vi "Autonomous.vi"() -> ()   [LabVIEW 2018]
uses:
  <vilib>/Studica/Studica Toolkit/Background/DIO Channel.ctl
  <vilib>/Studica/Studica Toolkit/Background/Mxp Selection.ctl
  <vilib>/robotics/Steering/Steering Frame/Apply Steering Frame Velocity to Motors.vi
  <vilib>/robotics/Steering/Steering Frame/Get Steering Frame Velocity from Motors.vi
  <vilib>/robotics/Steering/Steering Frame/NI_Robotics_Steering Frame.lvclass
  <vilib>/Studica/Studica Blackhawk/Blackhawk.lvlib
  <vilib>/Studica/Studica Toolkit/Background/I2C Channel.ctl
  <vilib>/Studica/Studica Toolkit/NavX/NavX.lvlib
panel:
  in  "Start Location (X,Y)":cluster{"X":dbl, "Y":dbl, "Theta":dbl}
  in  "Workstations":T1
  in  "Movement Accuracy":dbl=0.05 format="%#_13g"
  in  "SetPoints":T2
  in  "y":dbl=0.158982 format="%#_13g"
  in  "Speed":dbl[](array[numeric])=[-0.058732406271419055, -0.1288548481696414, 1.6548681508478632e-17]
  out "Hoist Height":dbl
  in  "CC's":T3={"CC 1"={"Ball #1"="Yellow", "Ball #2"="Red"}}
  in  "Wanted Location":dbl[](array[numeric])=[0.0, 0.0, 0.0]
  in  "Yellow Ball Bin":cluster{"X":dbl, "Y":dbl, "Theta":dbl}={"X"=-5.0, "Y"=5.0, "Theta"=0.0}
  in  "Orange Ball Bin":cluster{"X":dbl, "Y":dbl, "Theta":dbl}={"X"=5.0, "Y"=-5.0, "Theta"=0.0}
  in  "Red Ball Bin":cluster{"X":dbl, "Y":dbl, "Theta":dbl}={"X"=-5.0, "Y"=-5.0, "Theta"=0.0}
  in  "Blue Ball Bin":cluster{"X":dbl, "Y":dbl, "Theta":dbl}={"X"=5.0, "Y"=5.0, "Theta"=0.0}
  in  "CC 6":cluster{"X":dbl, "Y":dbl, "Theta":dbl}
  in  "CC 5":cluster{"X":dbl, "Y":dbl, "Theta":dbl}
  in  "CC 4":cluster{"X":dbl, "Y":dbl, "Theta":dbl}
  in  "CC 3":cluster{"X":dbl, "Y":dbl, "Theta":dbl}
  in  "CC 2":cluster{"X":dbl, "Y":dbl, "Theta":dbl}
  in  "CC 1":cluster{"X":dbl, "Y":dbl, "Theta":dbl}
  in  "Main Operation":string="Put Balls on CC"
  in  "Location PID":T4(array[cluster])=[{"proportional gain (Kc)"=10.0, "integral time (Ti, min)"=0.0, "derivative time (Td, min)"=0.0}, {"proportional gain (Kc)"=10.0, "integral time (Ti, min)"=0.0, "derivative time (Td, min)"=0.0}, {"proportional gain (Kc)"=10.0, "integral time (Ti, min)"=0.0, "derivative time (Td, min)"=0.0}] {"integral time (Ti, min)" min=0.0 step=0.0001}
  out "Estimated Robot Location":dbl[](array[numeric])=[0.036942802500546636, 0.08104996047957719, -1.0409154186309538e-17]
  out "Yaw":dbl
  in  "Wanted Rotation Angle":dbl[](array[numeric])=[0.0] format="%.2f"
  in  "NavX PID gains":T4(array[cluster])=[{"proportional gain (Kc)"=0.15, "integral time (Ti, min)"=0.0, "derivative time (Td, min)"=0.003}] {"integral time (Ti, min)" min=0.0 step=0.0001}
  in  "Hoist Setpoint (Height)":dbl
  in  "Button LED":bool
  out "estimated steering frame velocity":dbl[](array[numeric])
  in  "Green LED":bool=TRUE
  in  "Red LED":bool
  in  "Program Done?":bool
  in  "Robot Model":string(combo)="3-wheeled"
  in  "Reset Encoders":bool
  in  "StopMotors":bool
  in  "Stop Program":bool
  in  "Robot Facing":i16=4
  out "PID-Output":dbl[](array[numeric])=[-0.01145281922292672, 0.027486766135024127, -0.016033946912097405, -0.016033946912097405]
  in  "PID gains":T4(array[cluster])=[{"proportional gain (Kc)"=1.3, "integral time (Ti, min)"=0.004, "derivative time (Td, min)"=0.0}, {"proportional gain (Kc)"=1.3, "integral time (Ti, min)"=0.004, "derivative time (Td, min)"=0.0}, {"proportional gain (Kc)"=1.3, "integral time (Ti, min)"=0.004, "derivative time (Td, min)"=0.0}] {"proportional gain (Kc)" step=0.01; "integral time (Ti, min)" min=0.0 step=0.0001; "derivative time (Td, min)" step=0.0001}
  out "Actual-SpeedList":dbl[](array[numeric])
  in  "Linear Hoist":dbl(slide) scale=-1.0..1.0
  # "Configuration"
  # "LED's"
  # "Speed related shit"
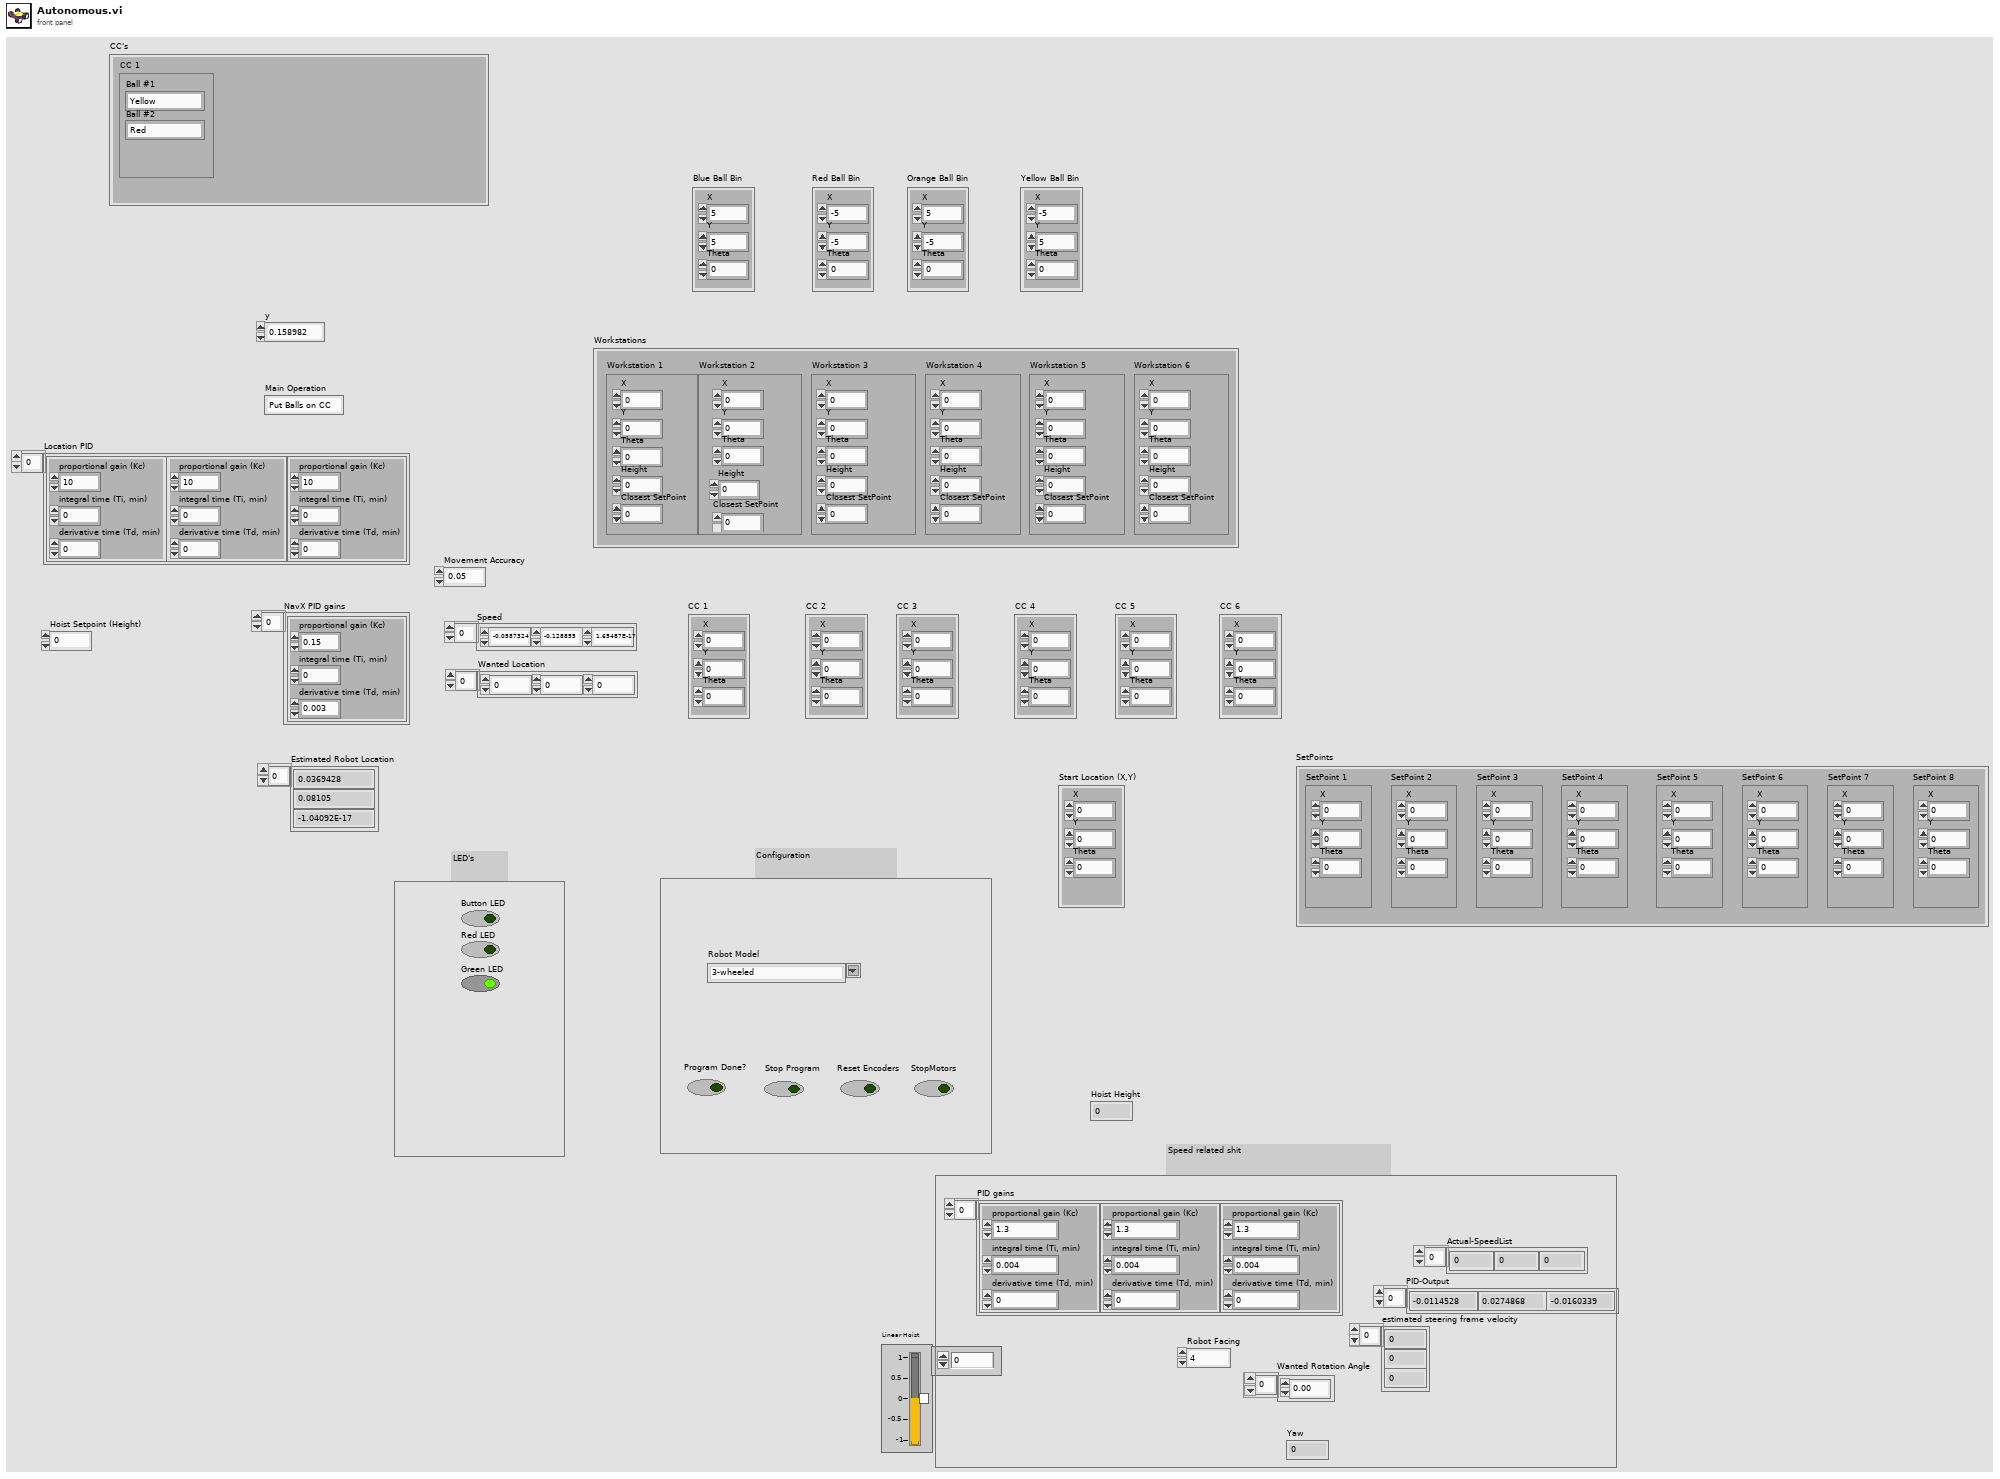
[diagram p1: front panel]
types:
  T1 = cluster{"Workstation 1":cluster{"X":dbl, "Y":dbl, "Theta":dbl, "Height":dbl, "Closest SetPoint":dbl}, "Workstation 2":cluster{"X":dbl, "Y":dbl, "Theta":dbl, "Height":dbl, "Closest SetPoint":dbl}, "Workstation 3":cluster{"X":dbl, "Y":dbl, "Theta":dbl, "Height":dbl, "Closest SetPoint":dbl}, "Workstation 4":cluster{"X":dbl, "Y":dbl, "Theta":dbl, "Height":dbl, "Closest SetPoint":dbl}, "Workstation 5":cluster{"X":dbl, "Y":dbl, "Theta":dbl, "Height":dbl, "Closest SetPoint":dbl}, "Workstation 6":cluster{"X":dbl, "Y":dbl, "Theta":dbl, "Height":dbl, "Closest SetPoint":dbl}}
  T2 = cluster{"SetPoint 1":cluster{"X":dbl, "Y":dbl, "Theta":dbl}, "SetPoint 2":cluster{"X":dbl, "Y":dbl, "Theta":dbl}, "SetPoint 3":cluster{"X":dbl, "Y":dbl, "Theta":dbl}, "SetPoint 4":cluster{"X":dbl, "Y":dbl, "Theta":dbl}, "SetPoint 5":cluster{"X":dbl, "Y":dbl, "Theta":dbl}, "SetPoint 6":cluster{"X":dbl, "Y":dbl, "Theta":dbl}, "SetPoint 7":cluster{"X":dbl, "Y":dbl, "Theta":dbl}, "SetPoint 8":cluster{"X":dbl, "Y":dbl, "Theta":dbl}}
  T3 = cluster{"CC 1":cluster{"Ball #1":string, "Ball #2":string}}
  T4 = cluster{"proportional gain (Kc)":dbl, "integral time (Ti, min)":dbl, "derivative time (Td, min)":dbl}[]
  T5 = typedef "DIO Channel.ctl" = enum16{"Not Connected", "A/DIO1", "A/DIO2", "A/DIO3", "A/DIO4", "A/DIO5", "A/DIO6", "A/DIO7", "A/DIO13", "B/DIO1", "B/DIO2", "B/DIO3", "B/DIO4", "B/DIO5", "B/DIO6", "B/DIO7", "B/DIO13", "C/DIO0", "C/DIO1", "C/DIO2", "C/DIO3", "C/DIO4", "C/DIO5", "C/DIO6", "C/DIO7"}
  T6 = typedef "Mxp Selection.ctl" = enum16{"MXP A", "MXP B"}
  T7 = typedef "I2C Channel.ctl" = enum16{"Not Connected", "A", "B"}
  T8 = cluster{"DIO Channel":T5, "FPGA VI Reference Out":refnum<k20>}
  T9 = typedef "I2C.lvlib/I2C Reference.ctl" = cluster{"myRIO Reference":T10, "I2C Channels Enum":T14, "I2C Configuration":T15}
  T10 = typedef "myRIO Generic Hardware Reference.ctl" = cluster{"myRIO Model":T11, "myRIO Hardware Reference":T12}
  T11 = typedef "Hardware Version Enum.ctl" = enum16{"Unknown", "myRIO-1900", "myRIO-1950", "roboRIO", "NI ELVIS RIO CM", "ELVIS III"}
  T12 = typedef "myRIO v1.0 Reference.ctl" = cluster{"Generic FPGA Reference":T13, "Allow multiple opens":bool}
  T13 = typedef "Generic FPGA Reference.ctl" = refnum<k20>
  T14 = typedef "I2C Channels Enum.ctl" = enum16{"Not Connected", "A/I2C", "B/I2C", "I2C/I2C"}
  T15 = typedef "I2C.lvlib/I2C Configuration.ctl" = cluster{"I2C Transfer Rate":T16}
  T16 = typedef "I2C.lvlib/I2C Transfer Rate.ctl" = enum16{"Standard mode (100 kbps)", "Fast mode (400 kbps)"}
  T17 = cluster{"I2C Ref Out":cluster{"I2C Channel":T7, "FPGA VI Reference Out":refnum<k20>}, "Connected":bool, "Slave Address (7-bit)":u8, "Registry":u8[]}
  T18 = cluster{"Yaw":dbl, "Roll":dbl, "Pitch":dbl, "Heading":dbl, "Fused Heading":dbl}
  T19 = cluster{"X":dbl, "Y":dbl, "Theta":dbl, "Height":dbl, "Closest SetPoint":dbl}[]
  T20 = cluster{"X":dbl, "Y":dbl, "Theta":dbl, "Height":dbl, "Closest SetPoint":dbl}
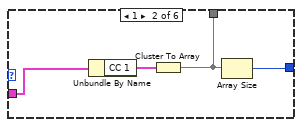
[diagram p3: hidden frame]
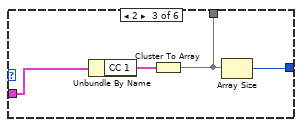
[diagram p4: hidden frame]
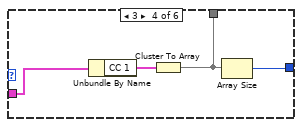
[diagram p5: hidden frame]
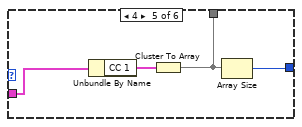
[diagram p6: hidden frame]
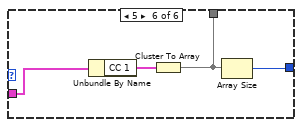
[diagram p7: hidden frame]
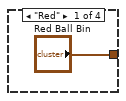
[diagram p8: hidden frame]
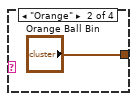
[diagram p9: hidden frame]
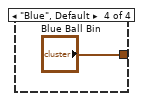
[diagram p10: hidden frame]
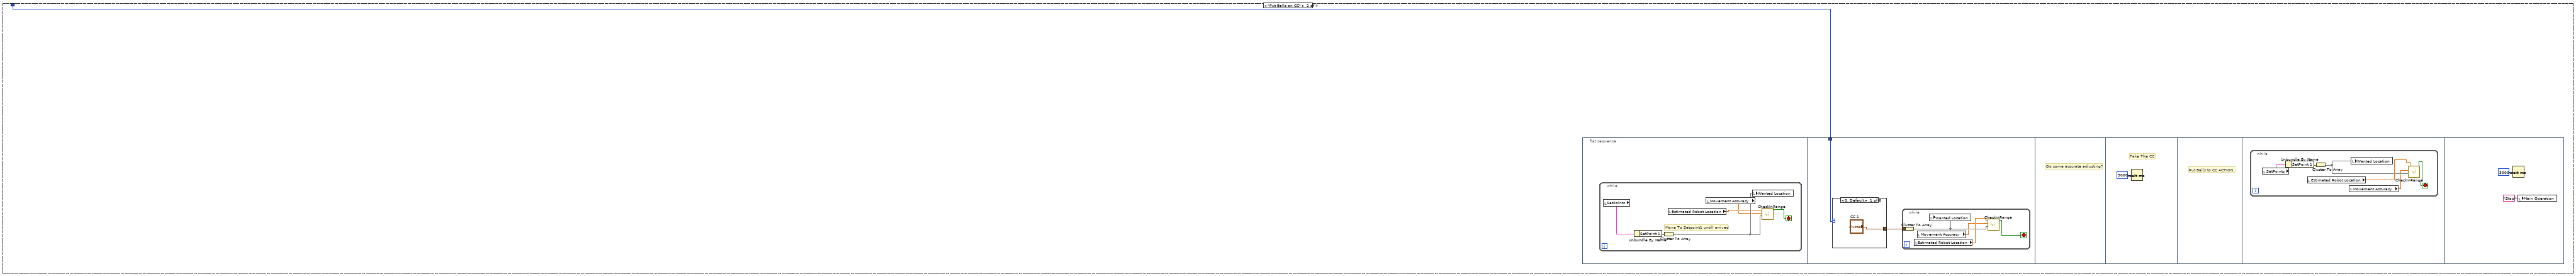
[diagram p12: hidden frame]
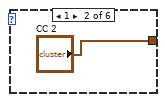
[diagram p13: hidden frame]
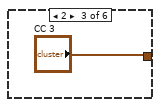
[diagram p14: hidden frame]
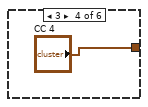
[diagram p15: hidden frame]
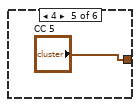
[diagram p16: hidden frame]
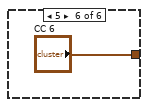
[diagram p17: hidden frame]
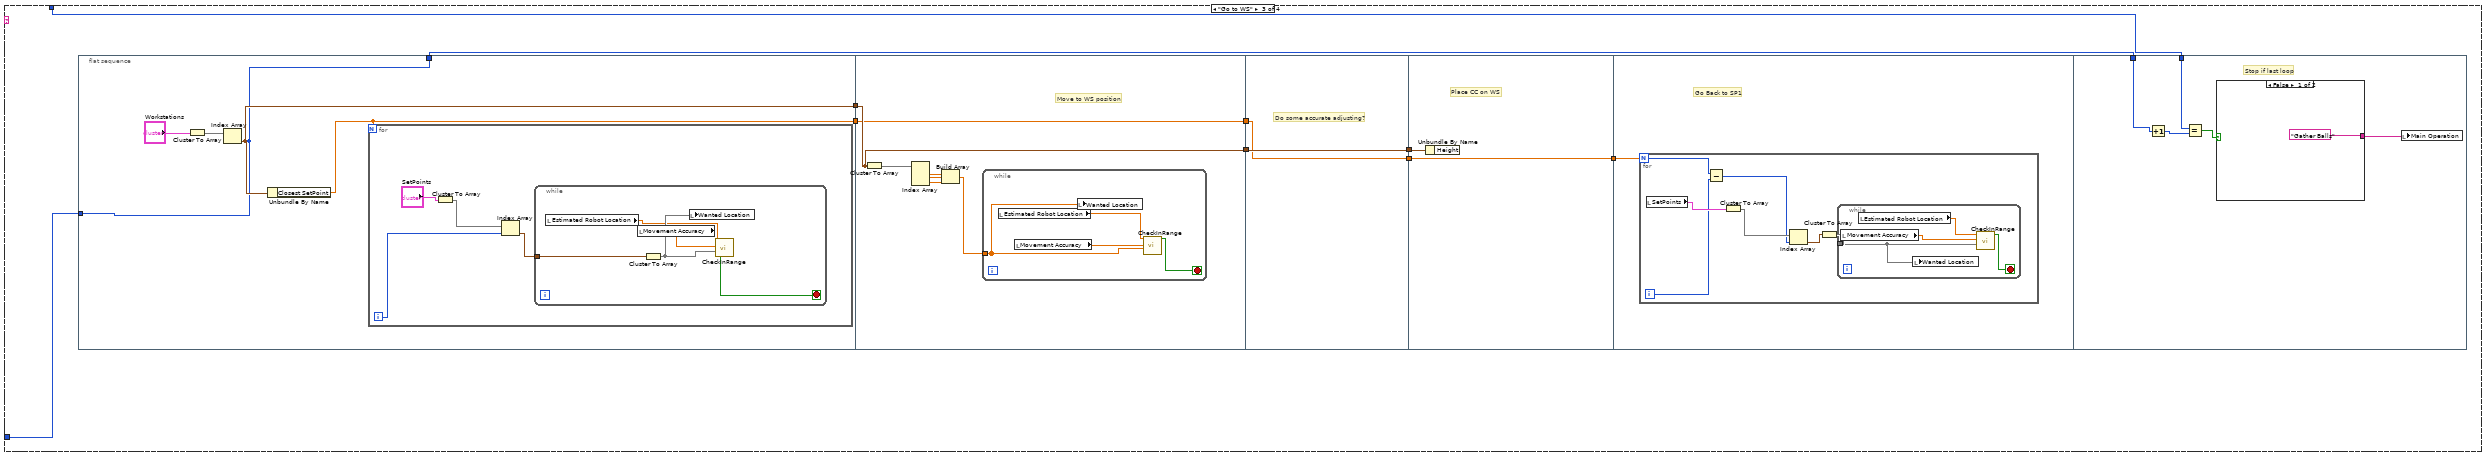
[diagram p18: hidden frame]
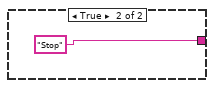
[diagram p19: hidden frame]
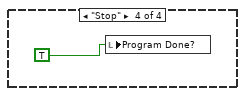
[diagram p20: hidden frame]
diagram:
  n1 = flat-sequence {
    frame #0 {
      # "Initialize"
      n2 = flat-sequence {
        frame #0 {
          w6 = FALSE ("StopMotors")
          w5 = FALSE ("StopMotors")
          n3 = flat-sequence {
            frame #0 {
              w7 = TRUE
              n4 = call <vilib>:"2 Encoders.vi"("Mxp Side"=Mxp_Selection."MXP A", "Reset Encoder 0"=w7, "Reset Encoder 1"=w7) -> ()  [unwired: 22 in, 3 out]
              n5 = call <vilib>:"2 Encoders.vi"("Mxp Side"=Mxp_Selection."MXP B", "Reset Encoder 0"=w7, "Reset Encoder 1"=w7) -> ()  [unwired: 22 in, 3 out]
            }
            frame #1 {
              w10 = FALSE
              n6 = call <vilib>:"2 Encoders.vi"("Mxp Side"=Mxp_Selection."MXP A", "Reset Encoder 0"=w10, "Reset Encoder 1"=w10) -> ()  [unwired: 22 in, 3 out]
              n7 = call <vilib>:"2 Encoders.vi"("Mxp Side"=Mxp_Selection."MXP B", "Reset Encoder 0"=w10, "Reset Encoder 1"=w10) -> ()  [unwired: 22 in, 3 out]
            }
          }
          n8 = local write "Button LED"(w6) -> ()
          n9 = local write "Red LED"(w6) -> ()
          n10 = local write "Green LED"(w6) -> ()
          n11 = local write "Program Done?"(w5) -> ()
          n12 = local write "Stop Program"(w5) -> ()
          n13 = local write "StopMotors"(w5) -> ()
          n14 = local write "Main Operation"("Gather Balls" ("Operation")) -> ()
        }
        frame #1 {
          n15 = disable-structure shown="Disabled" {
            frame Disabled {
              n16 = call <vilib>:"DIO Open.vi"("error in (no error)"=errorcluster {"status"=FALSE, "code"=0, "source"=""}, "DIO Channel"=DIO_Channel."C/DIO3") -> ("error out"=w16:errorcluster, "DIO Info Out"=w17:T8)  [unwired: 8 in]
              n17 = while {
                tunnel: w17 -> [w24]
                tunnel: w16 -> [w23]
                tunnel: [w22] -> w14
                tunnel: [w21] -> w13
                stop <- w19 stop-if-true
                # "Light Buttons LED"
                n18 = local write "Button LED"(TRUE ("Button LED")) -> ()
                n19 = call <vilib>:"C DIO Read.vi"("error in (no error)"=w23, "DIO Info In in"=w24) -> ("error out"=w21:errorcluster, "IN"=w19:bool, "DIO Info In out"=w22:T8)  [unwired: 7 in]
              }
              n20 = call <vilib>:"DIO Close.vi"("error in (no error)"=w13, "DIO Info In"=w14) -> ()  [unwired: 9 in, 1 out]
            }
            frame Enabled {
            }
          }
        }
        frame #2 {
          # "Light Green Led"
          n21 = local write "Button LED"(FALSE ("Button LED")) -> ()
          n22 = local write "Green LED"(TRUE ("Green LED")) -> ()
        }
      }
    }
    frame #1 {
      # "Loop for each cluster element(CC)"
      # "ENABLE THIS"
      # "Main"
      n23 = while {
        stop <- w205 stop-if-true
        n24 = local read "Estimated Robot Location"() -> (w199:dbl[])
        n25 = Multiply(x="Wanted Location", y="y") -> (x*y=w200:dbl[])
        n26 = Multiply(x=w199, y="y") -> (x*y=w197:dbl[])
        n27 = call "PID_array.vi"("output range"=cluster{"output high":dbl, "output low":dbl}[] [{"output high"=1.0, "output low"=-1.0}], "PID gains"="Location PID", "process variable"=w197, "setpoint"=w200) -> ("output"=w202:dbl[])  [unwired: 6 in, 1 out]
        n28 = local read "Stop Program"() -> (w205:bool)
        n29 = local write "Speed"(w202) -> ()
      }
      n30 = while {
        stop <- FALSE stop-if-true
        n31 = case shown="True" "Program Done?" {
          frame False {
          }
          frame True {
            # "Shut down Green Led"
            # "Light Red Led"
            n32 = local write "StopMotors"(TRUE ("StopMotors")) -> ()
            n33 = local write "Green LED"(FALSE ("Green LED")) -> ()
            n34 = local write "Red LED"(TRUE ("Red LED")) -> ()
          }
        }
      }
      n35 = disable-structure shown="Disabled" {
        frame Disabled {
          n36 = while {
            tunnel: tag "A/I2C" ("Channel Name") -> [w213]
            stop <- w212 stop-if-true
            n37 = call <vilib>:"Blackhawk i2c Open.vi"("error in (no error)"=errorcluster {"status"=FALSE, "code"=0, "source"=""}, "Channel Name"=w213) -> ("error out"=w209:errorcluster, "I2C Ref Out"=w210:T9)  [unwired: 2 in]
            n38 = local read "Stop Program"() -> (w212:bool)
            n39 = call <vilib>:"Blackhawk Relay.vi"("error in (no error)"=w209, "I2C Ref In"=w210) -> ("error out"=w207:errorcluster, "I2C Ref Out"=w208:T9)  [unwired: 8 in]
            n40 = call <vilib>:"Blackhawk DIO Read.vi"("I2C Ref In"=w208, "error in (no error)"=w207) -> ()  [unwired: 4 in, 3 out]
          }
        }
        frame Enabled {
        }
      }
      n41 = while {
        stop <- w222 stop-if-true
        n42 = local read "Hoist Height"() -> (w214:dbl)
        n43 = Multiply(x="Hoist Setpoint (Height)", y=45.382795) -> (x*y=w216:dbl)
        n44 = Multiply(x=w214, y=45.382795) -> (x*y=w220:dbl)
        n45 = Build Array(w216) -> (w217:dbl[])
        n46 = Build Array(w220) -> (w225:dbl[])
        n47 = call "PID_array.vi"("output range"=cluster{"output high":dbl, "output low":dbl}[] [{"output high"=1.0, "output low"=-1.0}], "process variable"=w225, "setpoint"=w217) -> ("output"=w224:dbl[])  [unwired: 7 in, 1 out]
        n48 = Index Array(array=w224) -> (element=w223:dbl)  [unwired: 1 in]
        n49 = local write "Linear Hoist"(w223) -> ()
        n50 = local read "Stop Program"() -> (w222:bool)
      }
      n51 = disable-structure shown="Disabled" {
        frame Disabled {
          n52 = while {
            tunnel: I2C_Channel."A" ("I2C Channel") -> [w195]
            stop <- w186 stop-if-true
            n53 = call <vilib>:"NavX Open.vi"("I2C Channel"=w195) -> ("NavX Info"=w196:T17)  [unwired: 9 in, 1 out]
            n54 = call <vilib>:"YRPHfH.vi"("NavX Info In"=w196) -> ("YRPHfH"=w191:T18)  [unwired: 3 in, 1 out]
            n55 = Unbundle By Name(w191) -> ("Yaw"=w190:dbl)
            "Yaw" <- w190
            n56 = Build Array(w190) -> (w189:dbl[])
            n57 = call "PID_array.vi"("output range"=cluster{"output high":dbl, "output low":dbl}[] [{"output high"=0.5, "output low"=-0.5}], "PID gains"="NavX PID gains", "process variable"=w189, "setpoint"="Wanted Rotation Angle") -> ("output"=w194:dbl[])  [unwired: 6 in, 1 out]
            n58 = Index Array(array=w194) -> (element=w187:dbl)  [unwired: 1 in]
            n59 = local read "Stop Program"() -> (w186:bool)
            n60 = local write item#-1(w187) -> ()
          }
        }
        frame Enabled {
        }
      }
      n61 = while "Motor Communication Loop" {
        stop <- w279 stop-if-true
        n62 = while {
          stop <- w280 stop-if-true
          n63 = case shown="False" "StopMotors" {
            frame False {
              n64 = while {
                tunnel: Mxp_Selection."MXP A" ("Mxp Side") -> [w295]
                tunnel: Mxp_Selection."MXP B" ("Mxp Side") -> [w294]
                stop <- w292 stop-if-true
                w291 = 50.0 ("Frequency [Hz]")
                n65 = local read "PID-Output"() -> (w293:dbl[])
                n66 = Index Array(array=w293) -> (element #1=w287:dbl, element #2=w286:dbl, element #3=w285:dbl)  [unwired: 3 in]
                n67 = local read "StopMotors"() -> (w292:bool)
                n68 = call <vilib>:"2 Motor.vi"("Mxp Side"=w294, "Speed M0"=w285, "Invert M0"=FALSE, "Speed M1"="Linear Hoist", "Frequency [Hz]"=w291) -> ()  [unwired: 14 in, 1 out]
                n69 = call <vilib>:"2 Motor.vi"("Mxp Side"=w295, "Speed M0"=w287, "Invert M0"=FALSE, "Speed M1"=w286, "Invert M1"=TRUE ("Invert M0"), "Frequency [Hz]"=w291) -> ()  [unwired: 13 in, 1 out]
              }
            }
            frame True {
              w296 = 50.0 ("Frequency [Hz]")
              w297 = 0.0 ("Speed M0")
              n70 = call <vilib>:"2 Motor.vi"("Mxp Side"=Mxp_Selection."MXP A", "Speed M0"=w297, "Speed M1"=w297, "Frequency [Hz]"=w296) -> ()  [unwired: 15 in, 1 out]
              n71 = call <vilib>:"2 Motor.vi"("Mxp Side"=Mxp_Selection."MXP B", "Speed M0"=w297, "Speed M1"=w297, "Frequency [Hz]"=w296) -> ()  [unwired: 15 in, 1 out]
            }
          }
          n72 = local read "Stop Program"() -> (w280:bool)
        }
        n73 = local read "Stop Program"() -> (w279:bool)
      }
      n74 = while "Wheel Velocity Measurement loop" {
        shift-right: [w235] -> _
        shift-left: _ -> [w254]
        shift-right: [w251] -> _
        shift-left: _ -> [w252]
        stop <- w247 stop-if-true
        w249 = 4.0 ("Wheel Diameter M1 (inches)")
        w257 = u32 1440 ("Ticks Per Rev M0")
        # "1440 * 3 * 10"
        # "Ticks travelled"
        # "Distance travelled\n(inch)"
        # "Wheel diam.\n(inch)"
        # "Ticks/rev"
        # "Ticks elapsed"
        # "Time elapsed"
        # "m/s"
        n75 = Wait (ms)(milliseconds to wait=u32 30) -> ()  [unwired: 1 out]
        n76 = call <vilib>:"2 Encoders.vi"("Mxp Side"=Mxp_Selection."MXP A", "Ticks Per Rev M0"=w257, "Wheel Diameter M0 (inches)"=w249, "Reset Encoder 0"="Reset Encoders", "Ticks Per Rev M1"=w257, "Wheel Diameter M1 (inches)"=w249, "Reset Encoder 1"="Reset Encoders") -> ("Distance M0 (inches)"=w258:dbl, "Distance M1 (inches)"=w259:dbl)  [unwired: 18 in, 1 out]
        n77 = call <vilib>:"2 Encoders.vi"("Mxp Side"=Mxp_Selection."MXP B", "Ticks Per Rev M0"=w257, "Wheel Diameter M0 (inches)"=w249, "Reset Encoder 0"="Reset Encoders", "Ticks Per Rev M1"=w257, "Wheel Diameter M1 (inches)"=w249, "Reset Encoder 1"="Reset Encoders") -> ("Distance M0 (inches)"=w260:dbl, "Distance M1 (inches)"=w250:dbl)  [unwired: 18 in, 1 out]
        n78 = Build Array(w258, w259, w260, w250) -> (w262:dbl[])
        n79 = local read "Robot Facing"() -> (w246:i16)
        n80 = Multiply(x=w262, y=2.54) -> (x*y=w236:dbl[])
        n81 = call "SteeringFrame.vi"() -> ("NI_Robotics_Steering Frame out"=w245:refnum<class "NI_Robotics_Steering Frame.lvclass">)  [unwired: 11 in]
        n82 = Multiply(x=w236, y=45.382795) -> (x*y=w235:dbl[])
        n83 = Tick Count (ms)() -> (millisecond timer value=w251:u32)
        n84 = case shown="2, Default" w246 {
          tunnel: w236 -> [w268 w274]
          tunnel: w245 -> [w267 w272]
          tunnel: [w265 w273] -> w243
          frame 4 {
            n85 = Build Array(0, 1, 2) -> (w266:i32[])
            n86 = call-poly <vilib>:"Get Velocity from Motors.vi"("wheel indexes"=w266, "ccw motor velocity states"=w268, "steering frame in"=w267) -> ("estimated steering frame velocity"=w265:dbl[])  [unwired: 6 in, 2 out]
          }
          frame 2, Default {
            n87 = Build Array(1, 2, 0) -> (w275:i32[])
            n88 = call-poly <vilib>:"Get Velocity from Motors.vi"("wheel indexes"=w275, "ccw motor velocity states"=w274, "steering frame in"=w272) -> ("estimated steering frame velocity"=w273:dbl[])  [unwired: 6 in, 2 out]
          }
        }
        n89 = Subtract(x=w235, y=w254) -> (x-y=w253:dbl[])
        n90 = Index Array(array=w235, index=3) -> (element=w233:dbl)
        n91 = Subtract(x=w251, y=w252) -> (x-y=w264:u32)
        n92 = Divide(x=w233, y=43.2) -> (x/y=→"Hoist Height":dbl)
        n93 = Cluster To Array(cluster="Start Location (X,Y)") -> (array=w244:dbl[])
        n94 = Divide(x=w253, y=w264) -> (x/y=w240:dbl[])
        n95 = Add(x=w244, y=w243) -> (x+y=→"Estimated Robot Location":dbl[])
        n96 = Divide(x=w240, y=10.0) -> (x/y=→"Actual-SpeedList":dbl[])
        n97 = local read "Stop Program"() -> (w247:bool)
      }
      n98 = Flatten To String(anything="CC's") -> (data string=w28:string)  [unwired: 3 in, 2 out]
      n99 = String Length(string=w28) -> (length=w27:i32)
      n100 = case shown="\"3-wheeled\", Default" "Robot Model" {
        frame "3-wheeled", Default {
          n101 = call "SteeringFrame.vi"() -> ("NI_Robotics_Steering Frame out"=w300:refnum<class "NI_Robotics_Steering Frame.lvclass">)  [unwired: 11 in]
          n102 = while "Motor Control Loop" {
            shift-right: [w313] -> _
            shift-left: w300 -> [w308]
            stop <- "Stop Program" stop-if-true
            # "Wanted speeds"
            # "PID-Adjusted\nOutput to Motors"
            # "Motor Velocity\nReal Time"
            # "PID Max. \nOutputRange"
            # "PID Setpoint"
            n103 = case shown="2, Default" "Robot Facing" {
              tunnel: w308 -> [w324 w335]
              tunnel: [w320 w331] -> w313
              tunnel: [w318 w328] -> w303
              tunnel: [w315 w326] -> w305
              tunnel: "Speed" -> [w314 w325]
              frame 2, Default {
                n104 = Build Array(1, 2, 0) -> (w317:i32[])
                n105 = local read "Actual-SpeedList"() -> (w316:dbl[])
                n106 = call-poly <vilib>:"Apply Velocity to Motors.vi"("wheel indexes"=w317, "steering frame velocity"=w314, "steering frame in"=w324) -> ("ccw motor velocity setpoints"=w318:dbl[], "steering frame out"=w319:refnum<class "NI_Robotics_Steering Frame.lvclass">)  [unwired: 4 in, 3 out]
                n107 = call-poly <vilib>:"Get Velocity from Motors.vi"("wheel indexes"=w317, "ccw motor velocity states"=w316, "steering frame in"=w319) -> ("estimated steering frame velocity"=w315:dbl[], "steering frame out"=w320:refnum<class "NI_Robotics_Steering Frame.lvclass">)  [unwired: 6 in, 1 out]
              }
              frame 4 {
                n108 = Build Array(0, 1, 2) -> (w329:i32[])
                n109 = local read "Actual-SpeedList"() -> (w327:dbl[])
                n110 = call-poly <vilib>:"Apply Velocity to Motors.vi"("wheel indexes"=w329, "steering frame velocity"=w325, "steering frame in"=w335) -> ("ccw motor velocity setpoints"=w328:dbl[], "steering frame out"=w330:refnum<class "NI_Robotics_Steering Frame.lvclass">)  [unwired: 4 in, 3 out]
                n111 = call-poly <vilib>:"Get Velocity from Motors.vi"("wheel indexes"=w329, "ccw motor velocity states"=w327, "steering frame in"=w330) -> ("estimated steering frame velocity"=w326:dbl[], "steering frame out"=w331:refnum<class "NI_Robotics_Steering Frame.lvclass">)  [unwired: 6 in, 1 out]
              }
            }
            "estimated steering frame velocity" <- w305
            n112 = local read "Actual-SpeedList"() -> (w306:dbl[])
            n113 = Divide(x=w303, y=40.0 ("Wheel Diameter M1 (inches)")) -> (x/y=w302:dbl[])
            n114 = call "PID_array.vi"("output range"=cluster{"output high":dbl, "output low":dbl}[] [{"output high"=1.0, "output low"=-1.0}, {"output high"=1.0, "output low"=-1.0}, {"output high"=1.0, "output low"=-1.0}, {"output high"=1.0, "output low"=-1.0}], "PID gains"="PID gains", "process variable"=w306, "setpoint"=w302) -> ("output"=→"PID-Output":dbl[])  [unwired: 6 in, 1 out]
          }
        }
      }
      n115 = for {
        N: w27 -> [w32]
        i -> [w31]
        # "Which CC is getting delivered"
        n116 = case shown="\"Gather Balls\", Default" "Main Operation" {
          tunnel: w32 -> [w36 w97 w126 _]
          tunnel: w31 -> [_ _ w128 _]
          frame "Gather Balls", Default {
            # "REMEMBER TO CHANGE THESE"
            n117 = local read "CC's"() -> (w37:T3)
            n118 = case shown="0, Default" w36 {
              tunnel: w37 -> [w41 w44 w48 w52 w56 w60]
              tunnel: [w38 w43 w47 w51 w55 w59] -> w35
              tunnel: [w39 w42 w46 w50 w54 w58] -> w34
              frame 0, Default {
                n119 = Unbundle By Name(w41) -> ("CC 1"=w40:cluster{"Ball #1":string, "Ball #2":string})
                n120 = Cluster To Array(cluster=w40) -> (array=w39:string[])
                n121 = Array Size(array=w39) -> (size(s)=w38:i32)
              }
              frame 1 {
                n122 = Unbundle By Name(w44) -> ("CC 1"=w45:cluster{"Ball #1":string, "Ball #2":string})
                n123 = Cluster To Array(cluster=w45) -> (array=w42:string[])
                n124 = Array Size(array=w42) -> (size(s)=w43:i32)
              }
              frame 2 {
                n125 = Unbundle By Name(w48) -> ("CC 1"=w49:cluster{"Ball #1":string, "Ball #2":string})
                n126 = Cluster To Array(cluster=w49) -> (array=w46:string[])
                n127 = Array Size(array=w46) -> (size(s)=w47:i32)
              }
              frame 3 {
                n128 = Unbundle By Name(w52) -> ("CC 1"=w53:cluster{"Ball #1":string, "Ball #2":string})
                n129 = Cluster To Array(cluster=w53) -> (array=w50:string[])
                n130 = Array Size(array=w50) -> (size(s)=w51:i32)
              }
              frame 4 {
                n131 = Unbundle By Name(w56) -> ("CC 1"=w57:cluster{"Ball #1":string, "Ball #2":string})
                n132 = Cluster To Array(cluster=w57) -> (array=w54:string[])
                n133 = Array Size(array=w54) -> (size(s)=w55:i32)
              }
              frame 5 {
                n134 = Unbundle By Name(w60) -> ("CC 1"=w61:cluster{"Ball #1":string, "Ball #2":string})
                n135 = Cluster To Array(cluster=w61) -> (array=w58:string[])
                n136 = Array Size(array=w58) -> (size(s)=w59:i32)
              }
            }
            n137 = for {
              N: w35 -> [w62]
              tunnel: w34 -> [w63]
              i -> [w64]
              n138 = flat-sequence {
                tunnel: w64 -> [w74]
                tunnel: w63 -> [w72]
                tunnel: w64 -> [w95]
                tunnel: w62 -> [w92]
                frame #0 {
                  n139 = while {
                    stop <- w67 stop-if-true
                    # "Move To Setpoint1 untill arrived"
                    n140 = local read "SetPoints"() -> (w65:T2)
                    n141 = Unbundle By Name(w65) -> ("SetPoint 1"=w66:cluster{"X":dbl, "Y":dbl, "Theta":dbl})
                    n142 = Cluster To Array(cluster=w66) -> (array=w69:dbl[])
                    n143 = local read "Estimated Robot Location"() -> (w68:dbl[])
                    n144 = local write "Wanted Location"(w69) -> ()
                    n145 = call "CheckInRange"("SetPoint"=w69, "y"="Movement Accuracy", "Estimated Robot Location"=w68) -> ("Boolean"=w67:bool)  [unwired: 8 in]
                  }
                }
                frame #1 {
                  n146 = Index Array(array=w72, index=w74) -> (element=w71:string)
                  n147 = case shown="\"Yellow\"" w71 {
                    tunnel: ["Red Ball Bin" "Orange Ball Bin" "Yellow Ball Bin" "Blue Ball Bin"] -> w73
                    frame "Red" {
                    }
                    frame "Orange" {
                    }
                    frame "Yellow" {
                    }
                    frame "Blue", Default {
                    }
                  }
                  n148 = while {
                    tunnel: w73 -> [w79]
                    stop <- w76 stop-if-true
                    n149 = Cluster To Array(cluster=w79) -> (array=w77:dbl[])
                    n150 = local read "Estimated Robot Location"() -> (w78:dbl[])
                    n151 = local read "Movement Accuracy"() -> (w75:dbl)
                    n152 = local write "Wanted Location"(w77) -> ()
                    n153 = call "CheckInRange"("SetPoint"=w77, "y"=w75, "Estimated Robot Location"=w78) -> ("Boolean"=w76:bool)  [unwired: 8 in]
                  }
                }
                frame #2 {
                  # "PICKUP BALL"
                  n154 = Wait (ms)(milliseconds to wait=u32 3000) -> ()  [unwired: 1 out]
                }
                frame #3 {
                  n155 = while {
                    stop <- w89 stop-if-true
                    n156 = local read "SetPoints"() -> (w86:T2)
                    n157 = local read "Estimated Robot Location"() -> (w90:dbl[])
                    n158 = Unbundle By Name(w86) -> ("SetPoint 1"=w88:cluster{"X":dbl, "Y":dbl, "Theta":dbl})
                    n159 = local read "Movement Accuracy"() -> (w85:dbl)
                    n160 = Cluster To Array(cluster=w88) -> (array=w87:dbl[])
                    n161 = local write "Wanted Location"(w87) -> ()
                    n162 = call "CheckInRange"("SetPoint"=w87, "y"=w85, "Estimated Robot Location"=w90) -> ("Boolean"=w89:bool)  [unwired: 8 in]
                  }
                }
                frame #4 {
                  n163 = Decrement(x=w92) -> (x-1=w93:i32)
                  n164 = Equal?(x=w95, y=w93) -> (x = y?=w94:bool)
                  n165 = case shown="True" w94 {
                    frame False {
                    }
                    frame True {
                      n166 = local write "Main Operation"("Put Balls on CC" ("Main Operation")) -> ()
                    }
                  }
                  n167 = Wait (ms)(milliseconds to wait=u32 3000) -> ()  [unwired: 1 out]
                }
              }
            }
          }
          frame "Put Balls on CC" {
            n168 = flat-sequence {
              tunnel: w97 -> [w104]
              frame #0 {
                n169 = while {
                  stop <- w101 stop-if-true
                  # "Move To Setpoint1 untill arrived"
                  n170 = local read "SetPoints"() -> (w100:T2)
                  n171 = Unbundle By Name(w100) -> ("SetPoint 1"=w99:cluster{"X":dbl, "Y":dbl, "Theta":dbl})
                  n172 = Cluster To Array(cluster=w99) -> (array=w103:dbl[])
                  n173 = local read "Estimated Robot Location"() -> (w102:dbl[])
                  n174 = local read "Movement Accuracy"() -> (w98:dbl)
                  n175 = local write "Wanted Location"(w103) -> ()
                  n176 = call "CheckInRange"("SetPoint"=w103, "y"=w98, "Estimated Robot Location"=w102) -> ("Boolean"=w101:bool)  [unwired: 8 in]
                }
              }
              frame #1 {
                n177 = case shown="0, Default" w104 {
                  tunnel: ["CC 1" "CC 2" "CC 3" "CC 4" "CC 5" "CC 6"] -> w105
                  frame 0, Default {
                  }
                  frame 1 {
                  }
                  frame 2 {
                  }
                  frame 3 {
                  }
                  frame 4 {
                  }
                  frame 5 {
                  }
                }
                n178 = while {
                  tunnel: w105 -> [w114]
                  stop <- w115 stop-if-true
                  n179 = Cluster To Array(cluster=w114) -> (array=w113:dbl[])
                  n180 = local read "Estimated Robot Location"() -> (w116:dbl[])
                  n181 = local read "Movement Accuracy"() -> (w112:dbl)
                  n182 = local write "Wanted Location"(w113) -> ()
                  n183 = call "CheckInRange"("SetPoint"=w113, "y"=w112, "Estimated Robot Location"=w116) -> ("Boolean"=w115:bool)  [unwired: 8 in]
                }
              }
              frame #2 {
                # "Do some accurate adjusting?"
              }
              frame #3 {
                # "Take The CC"
                n184 = Wait (ms)(milliseconds to wait=u32 3000) -> ()  [unwired: 1 out]
              }
              frame #4 {
                # "Put Balls to CC ACTION"
              }
              frame #5 {
                n185 = while {
                  stop <- w122 stop-if-true
                  n186 = local read "SetPoints"() -> (w119:T2)
                  n187 = Unbundle By Name(w119) -> ("SetPoint 1"=w121:cluster{"X":dbl, "Y":dbl, "Theta":dbl})
                  n188 = local read "Estimated Robot Location"() -> (w123:dbl[])
                  n189 = Cluster To Array(cluster=w121) -> (array=w120:dbl[])
                  n190 = local read "Movement Accuracy"() -> (w118:dbl)
                  n191 = local write "Wanted Location"(w120) -> ()
                  n192 = call "CheckInRange"("SetPoint"=w120, "y"=w118, "Estimated Robot Location"=w123) -> ("Boolean"=w122:bool)  [unwired: 8 in]
                }
              }
              frame #6 {
                n193 = Wait (ms)(milliseconds to wait=u32 3000) -> ()  [unwired: 1 out]
                n194 = local write "Main Operation"("Stop" ("Main Operation")) -> ()
              }
            }
          }
          frame "Go to WS" {
            n195 = flat-sequence {
              tunnel: [w138] -> w135
              tunnel: [w137] -> w132
              tunnel: w128 -> [w136]
              tunnel: [w136] -> w127
              tunnel: w135 -> [w151]
              tunnel: [w151] -> w134
              tunnel: w132 -> [w150]
              tunnel: [w150] -> w131
              tunnel: w134 -> [w162]
              tunnel: [w162] -> w133
              tunnel: w131 -> [w161]
              tunnel: [w161] -> w130
              tunnel: w133 -> [w164]
              tunnel: w130 -> [w163]
              tunnel: [w163] -> w129
              tunnel: w129 -> [w165]
              tunnel: w127 -> [w180]
              tunnel: w126 -> [w181]
              frame #0 {
                n196 = Cluster To Array(cluster="Workstations") -> (array=w140:T19)
                n197 = Index Array(array=w140, index=w136) -> (element=w138:T20)
                n198 = Unbundle By Name(w138) -> ("Closest SetPoint"=w137:dbl)
                n199 = for {
                  N: w137 -> [_]
                  i -> [w141]
                  n200 = Cluster To Array(cluster="SetPoints") -> (array=w143:cluster{"X":dbl, "Y":dbl, "Theta":dbl}[])
                  n201 = Index Array(array=w143, index=w141) -> (element=w142:cluster{"X":dbl, "Y":dbl, "Theta":dbl})
                  n202 = while {
                    tunnel: w142 -> [w146]
                    stop <- w149 stop-if-true
                    n203 = local read "Estimated Robot Location"() -> (w145:dbl[])
                    n204 = local read "Movement Accuracy"() -> (w147:dbl)
                    n205 = Cluster To Array(cluster=w146) -> (array=w148:dbl[])
                    n206 = local write "Wanted Location"(w148) -> ()
                    n207 = call "CheckInRange"("SetPoint"=w148, "y"=w147, "Estimated Robot Location"=w145) -> ("Boolean"=w149:bool)  [unwired: 8 in]
                  }
                }
              }
              frame #1 {
                # "Move to WS position"
                n208 = Cluster To Array(cluster=w151) -> (array=w156:dbl[])
                n209 = Index Array(array=w156) -> (element #1=w155:dbl, element #2=w154:dbl, element #3=w153:dbl)  [unwired: 3 in]
                n210 = Build Array(w155, w154, w153) -> (w152:dbl[])
                n211 = while {
                  tunnel: w152 -> [w158]
                  stop <- w160 stop-if-true
                  n212 = local read "Estimated Robot Location"() -> (w157:dbl[])
                  n213 = local read "Movement Accuracy"() -> (w159:dbl)
                  n214 = local write "Wanted Location"(w158) -> ()
                  n215 = call "CheckInRange"("SetPoint"=w158, "y"=w159, "Estimated Robot Location"=w157) -> ("Boolean"=w160:bool)  [unwired: 8 in]
                }
              }
              frame #2 {
                # "Do some accurate adjusting?"
              }
              frame #3 {
                # "Place CC on WS"
                n216 = Unbundle By Name(w164) -> ()  [unwired: 1 out]
              }
              frame #4 {
                # "Go Back to SP1"
                n217 = for {
                  N: w165 -> [w170]
                  i -> [w169]
                  n218 = local read "SetPoints"() -> (w171:T2)
                  n219 = Subtract(x=w170, y=w169) -> (x-y=w168:i32)
                  n220 = Cluster To Array(cluster=w171) -> (array=w172:cluster{"X":dbl, "Y":dbl, "Theta":dbl}[])
                  n221 = Index Array(array=w172, index=w168) -> (element=w167:cluster{"X":dbl, "Y":dbl, "Theta":dbl})
                  n222 = Cluster To Array(cluster=w167) -> (array=w166:dbl[])
                  n223 = while {
                    tunnel: w166 -> [w175]
                    stop <- w174 stop-if-true
                    n224 = local read "Movement Accuracy"() -> (w173:dbl)
                    n225 = local read "Estimated Robot Location"() -> (w176:dbl[])
                    n226 = local write "Wanted Location"(w175) -> ()
                    n227 = call "CheckInRange"("SetPoint"=w175, "y"=w173, "Estimated Robot Location"=w176) -> ("Boolean"=w174:bool)  [unwired: 8 in]
                  }
                }
              }
              frame #5 {
                # "Stop if last loop"
                n228 = Increment(x=w180) -> (x+1=w179:i32)
                n229 = Equal?(x=w181, y=w179) -> (x = y?=w178:bool)
                n230 = case shown="False" w178 {
                  tunnel: ["Gather Balls" "Stop"] -> w177
                  frame False {
                  }
                  frame True {
                  }
                }
                n231 = local write "Main Operation"(w177) -> ()
              }
            }
          }
          frame "Stop" {
            n232 = local write "Program Done?"(TRUE) -> ()
          }
        }
      }
    }
  }
  n233 = while "LED loop" {
    tunnel: DIO_Channel."C/DIO1" ("DIO Channel") -> [w345]
    tunnel: DIO_Channel."C/DIO0" ("DIO Channel") -> [w342]
    tunnel: DIO_Channel."C/DIO2" ("DIO Channel") -> [w336]
    stop <- w340 stop-if-true
    n234 = call <vilib>:"DIO Open.vi"("DIO Channel"=w345) -> ("error out"=w347:errorcluster, "DIO Info Out"=w348:T8)  [unwired: 9 in]
    n235 = call <vilib>:"DIO Open.vi"("DIO Channel"=w342) -> ("error out"=w343:errorcluster, "DIO Info Out"=w344:T8)  [unwired: 9 in]
    n236 = local read "Stop Program"() -> (w340:bool)
    n237 = call <vilib>:"DIO Write.vi"("error in (no error)"=w347, "Input"="Green LED", "DIO Info In"=w348) -> ()  [unwired: 7 in, 2 out]
    n238 = call <vilib>:"DIO Write.vi"("error in (no error)"=w343, "Input"="Red LED", "DIO Info In"=w344) -> ()  [unwired: 7 in, 2 out]
    n239 = call <vilib>:"DIO Open.vi"("DIO Channel"=w336) -> ("error out"=w338:errorcluster, "DIO Info Out"=w339:T8)  [unwired: 9 in]
    n240 = call <vilib>:"DIO Write.vi"("error in (no error)"=w338, "Input"="Button LED", "DIO Info In"=w339) -> ()  [unwired: 7 in, 2 out]
  }
